vi "Pointer.Dispose.vi"(8 "error in (no error)":errorcluster, 11 "pointer":u64 format="%016x") -> (0 "error out":errorcluster, 3 "return":i32)   [LabVIEW 2016, in "VeriStand Data.lvlib"]
doc: "Disposes of the provided <B>pointer</B> that was allocated previously by the Pointer.New VI."
uses:
  VeriStand Data.lvlib
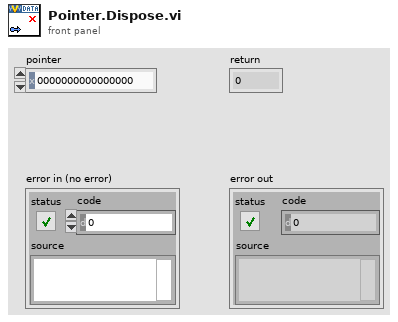
[diagram p1: front panel]
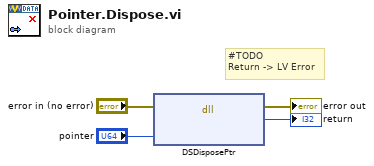
[diagram p0: block diagram]
diagram:
  # "#TODO\nReturn -> LV Error"
  n1 = dll-call lib="LabVIEW" fn="DSDisposePtr"(error in="error in (no error)", "ptr"="pointer") -> (error out=→"error out":errorcluster, "return"=→"return":i32)  [unwired: 3 in, 1 out]
